vi "Python convention.vi"(3 "String stream In":string="#This is a  .ini reader with Python comment style parser\n\n[DIOinterface] #Holds external Board interface\nPn4TO= 1300 # Pneumatic 1 output timeout in miliSeconds\nOptionPO= true #this enable pullUp Resistors when true\nLED23= 0xFF0000 #LED23 is a RGB LED , valid Values: RED, BLUE, GREEN, WHITE or HEX COLOR (RGB)\n\n[UILang]  #This holds all the language variables\nlang = 0 # valid values: 0 ->Finish , 1->English, 2->Spanish, 3->French, 4->Japanese, 5->German, 6->Hebrew\ngreeting = Plastilinapps, Tervetoula!! #Used for the main welcome page\ngreetingType= 1  # Valid Values 1=PopUp; 2=modal window\n\n[DBCon] #Database Credentials\nconType = 0 #Valid Values:  0->ODBC,  1->ADO (Connection String), 2->JDBC\nhost = MySQL #this is the host not the Database engine type\nuser= DataPub  #This a public username\npwd = 123 #this is a public password\n\n", 5 "error in":errorcluster) -> (23 "String parsed out":string, 25 "error out":errorcluster)   [LabVIEW 2015]
doc: "This VI parsed out the comments using the Pyhton comment convention.\ni.e:\nmyKey = myValue #myComment, this one is going to be parse-out\n\nDeveloped by Ezequiel Gonzalez plastilinapps.com"
panel:
  # "Developed by Ezequiel Gonzalez\nPlastilinapps.com  2015"
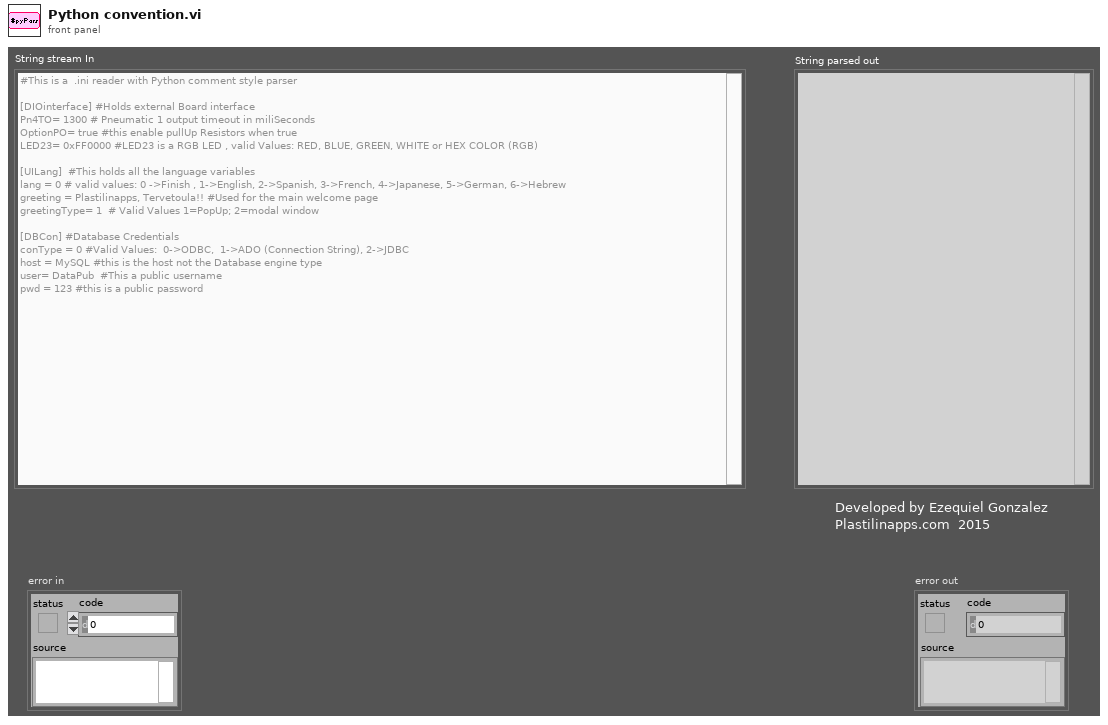
[diagram p1: front panel]
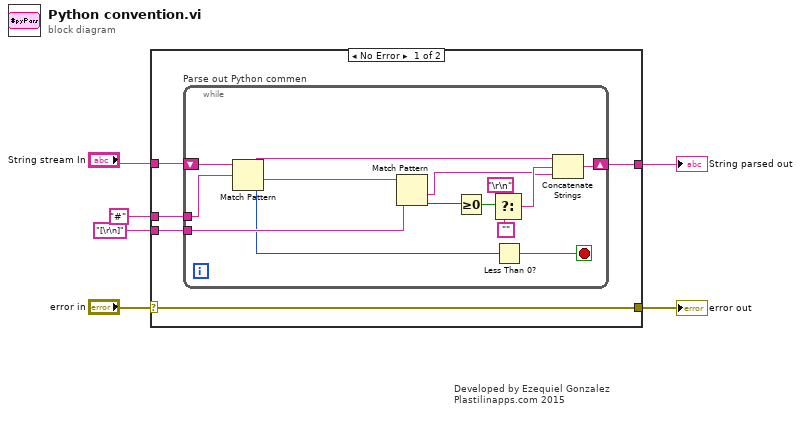
[diagram p0: block diagram]
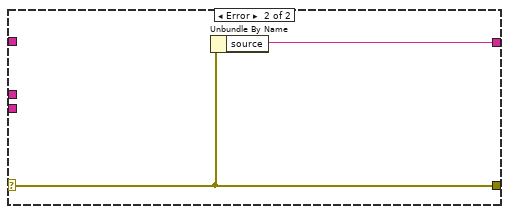
[diagram p2: hidden frame]
diagram:
  # "Developed by Ezequiel Gonzalez\nPlastilinapps.com 2015"
  n1 = case shown="No Error" "error in" {
    selector: "error in" -> [w7 w27]
    tunnel: "String stream In" -> [w11 _]
    tunnel: "#" ("regular expression") -> [w10 _]
    tunnel: "[\r\n]" ("regular expression") -> [w9 _]
    tunnel: [w8 w26] -> w2
    tunnel: [w7 w27] -> w1
    frame No Error {
      n2 = while "Parse out Python commen" {
        tunnel: w10 -> [w25]
        tunnel: w9 -> [w22]
        shift-right: [w19] -> w8
        shift-left: w11 -> [w13]
        stop <- w24 stop-if-true
        n3 = Match Pattern(string=w13, regular expression=w25) -> (before substring=w20:string, after substring=w23:string, offset past match=w21:i32)  [unwired: 1 in, 1 out]
        n4 = Match Pattern(string=w23, regular expression=w22) -> (after substring=w12:string, offset past match=w18:i32)  [unwired: 1 in, 2 out]
        n5 = Greater Or Equal To 0?(x=w18) -> (x >= 0?=w16:bool)
        n6 = Select(t="\r\n", s=w16, f="") -> (s? t:f=w14:string)
        n7 = Less Than 0?(x=w21) -> (x < 0?=w24:bool)
        n8 = Concatenate Strings(w20, w14, w12) -> (w19:string)
      }
    }
    frame Error {
      n9 = Unbundle By Name(w27) -> ("source"=w26:string)
    }
  }
  "String parsed out" <- w2
  "error out" <- w1
